vi "Get FK Exposure Time.vi"(8 "error in (no error)":errorcluster, 11 "time":sgl) -> (0 "error out":errorcluster, 2 "function return":u32, 3 "time out":sgl)   [LabVIEW 2014, in "atmcd32d.lvlib"]
doc: "unsigned int WINAPI GetFKExposureTime(float * time);"
uses:
  atmcd32d.lvlib
  atmcd32d.dll
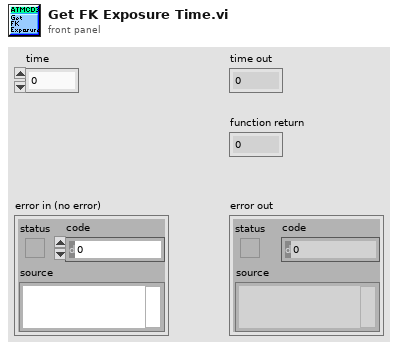
[diagram p1: front panel]
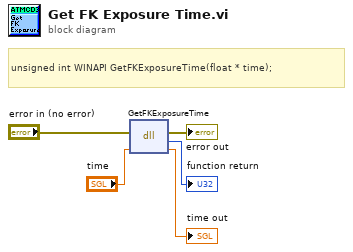
[diagram p0: block diagram]
diagram:
  # "unsigned int WINAPI GetFKExposureTime(float * time);"
  n1 = dll-call lib="C:/Users/Bakir/Documents/Lambda2-Testing/lib/Andorlib/atmcd32d.*" fn="GetFKExposureTime"(error in="error in (no error)", "time"="time") -> (error out=→"error out":errorcluster, →"function return":u32, "time"=→"time out":sgl)  [unwired: 2 in, 1 out]
